vi "Data_Decimate.vi"(5 "Decimate ?":bool, 7 "Is Mass ?":bool, 8 "error in (no error)":errorcluster, 10 "Dataset":cluster{sgl[], sgl[]}[](array[cluster]), 11 "GraphXY":refnum<vi>) -> (0 "error out":errorcluster)   [LabVIEW 2018]
doc: "This VI decimates the data for the GraphXY.\n- Checks the X-scale of the GraphXY, the size of the data, and the pixel size of the screen\n- If the size of the data to be diplayed is less than 1 million of pixels : do nothing\n- If the size of the data is too large for the current display, decimate the data\n- The decimation factor is function of the \"Points per Pixel\" multiplied by the size of the screen in pixels\n- The \"Points per Pixel\" value can be updated through the global variable \"GraphXY Points per Pixel\""
uses:
  Global_Variables.vi
panel:
  out "Number of Points Currently Displayed":i32
  out "Decimation Factor":u32
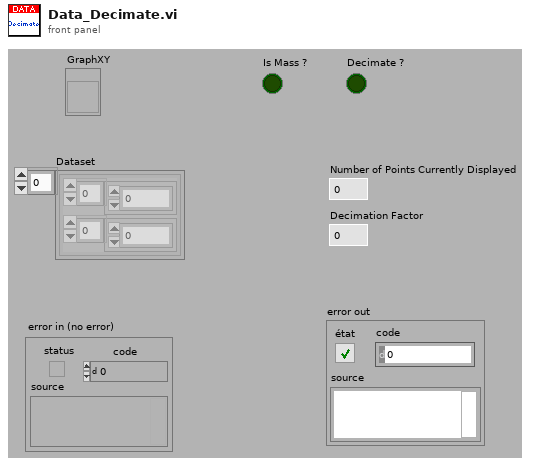
[diagram p1: front panel]
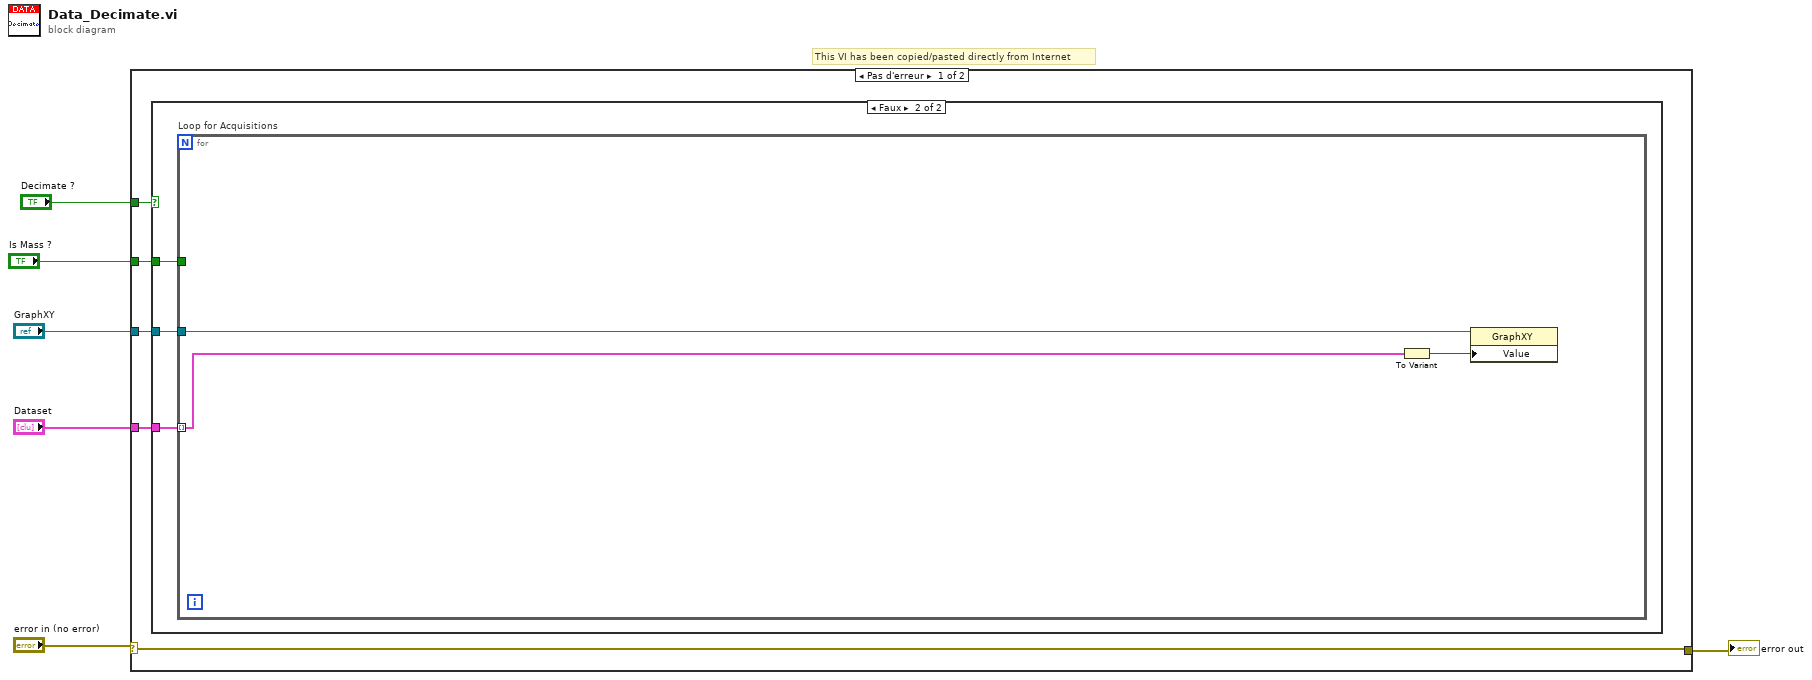
[diagram p0: block diagram]
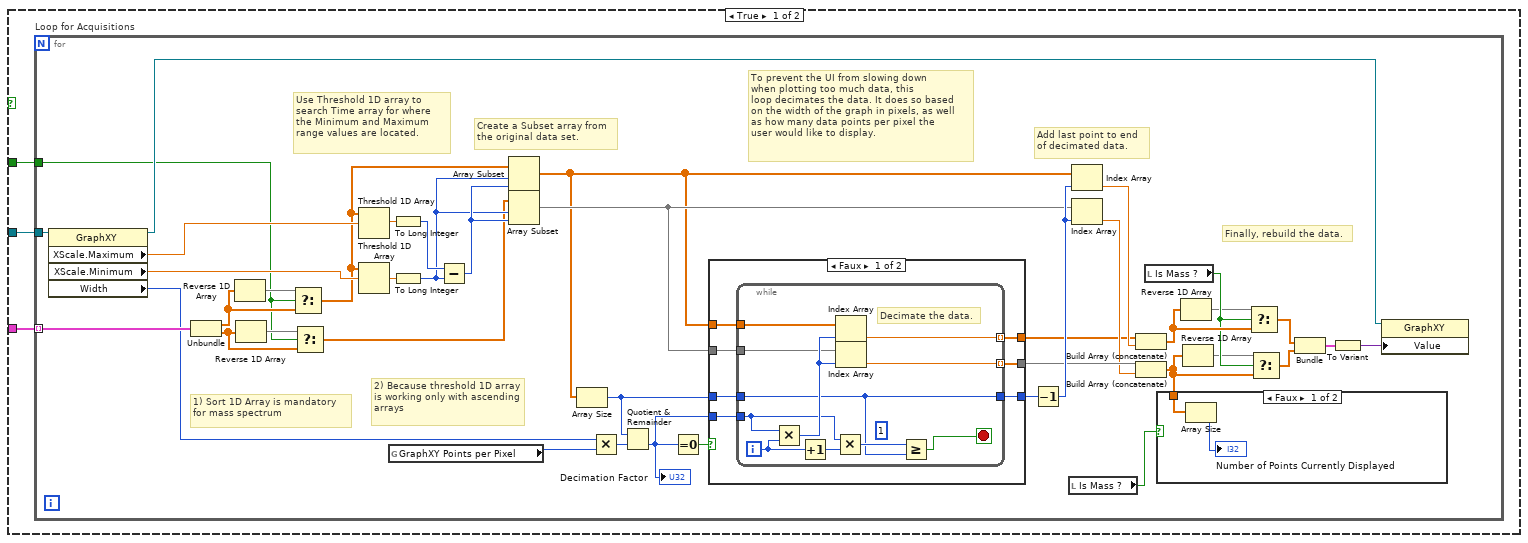
[diagram p2: hidden frame]
diagram:
  # "This VI has been copied/pasted directly from Internet"
  n1 = case shown="Pas d'erreur" "error in (no error)" {
    selector: "error in (no error)" -> [w9 w85]
    tunnel: [w9 w85] -> w5
    tunnel: "GraphXY" -> [w10 _]
    tunnel: "Dataset" -> [w11 _]
    tunnel: "Is Mass ?" -> [w8 _]
    tunnel: "Decimate ?" -> [w7 _]
    frame No Error {
      n2 = case shown="Faux" w7 {
        tunnel: w11 -> [w14 w81]
        tunnel: w10 -> [w13 w80]
        tunnel: w8 -> [w12 w79]
        frame True {
          n3 = for "Loop for Acquisitions" {
            tunnel: w14 -> [w55] mode=indexing
            tunnel: w13 -> [w54]
            tunnel: w12 -> [w23]
            # "1) Sort 1D Array is mandatory for mass spectrum"
            # "2) Because threshold 1D array is working only with ascending arrays"
            # "Add last point to end\nof decimated data."
            # "Finally, rebuild the data."
            # "To prevent the UI from slowing down\nwhen plotting too much data, this\nloop decimates the data. It does so based\non the width of the graph in pixels, as well\nas how many data points per pixel the\nuser would like to display."
            # "Create a Subset array from\nthe original data set."
            # "Use Threshold 1D array to\nsearch Time array for where\nthe Minimum and Maximum\nrange values are located."
            n4 = property class="GraphXY"(reference=w54) -> (reference out=w31:refnum<vi>, "XScale.Maximum"=w36:dbl, "XScale.Minimum"=w35:dbl, "Width"=w32:u32)  [unwired: 1 in, 1 out]
            n5 = Unbundle(w55) -> (w29:sgl[], w24:sgl[])
            n6 = Reverse 1D Array(array=w29) -> (reversed array=w28:sgl[])
            n7 = Reverse 1D Array(array=w24) -> (reversed array=w26:sgl[])
            n8 = Select(t=w28, s=w23, f=w29) -> (s? t:f=w27:sgl[])
            n9 = Select(t=w26, s=w23, f=w24) -> (s? t:f=w25:sgl[])
            n10 = Threshold 1D Array(2:w36, 3:w27) -> (0:w52:sgl)  [unwired: 1 in]
            n11 = Threshold 1D Array(2:w35, 3:w27) -> (0:w51:sgl)  [unwired: 1 in]
            n12 = global read "Global_Variables.vi" "GraphXY Points per Pixel"() -> (w30:i32)
            n13 = To Long Integer(number=w52) -> (32bit integer=w44:i32)
            n14 = To Long Integer(number=w51) -> (32bit integer=w43:i32)
            n15 = Subtract(x=w44, y=w43) -> (x-y=w53:i32)
            n16 = Array Subset(array=w27, index=w43, length=w53) -> (w38:sgl[])
            n17 = Array Subset(array=w25, index=w43, length=w53) -> (w48:sgl[])
            n18 = Array Size(array=w38) -> (size(s)=w42:i32)
            n19 = Multiply(x=w32, y=w30) -> (x*y=w39:u32)
            n20 = Quotient & Remainder(x=w42, y=w39) -> (floor(x/y)=w37:u32)  [unwired: 1 out]
            "Decimation Factor" <- w37
            n21 = Equal To 0?(x=w37) -> (x = 0?=w40:bool)
            n22 = case shown="Faux" w40 {
              tunnel: [w64 w76] -> w50
              tunnel: w38 -> [w63 w78]
              tunnel: w48 -> [w62 w77]
              tunnel: [w61 w77] -> w47
              tunnel: w42 -> [w60 w76]
              tunnel: [w59 w78] -> w41
              tunnel: w37 -> [w58 _]
              frame False {
                n23 = while {
                  tunnel: w63 -> [w72]
                  tunnel: w62 -> [w68]
                  tunnel: w60 -> [w66]
                  tunnel: [w70] -> w59 mode=indexing
                  tunnel: [w69] -> w61 mode=indexing
                  tunnel: w58 -> [w67]
                  tunnel: [w66] -> w64
                  i -> [w75]
                  stop <- w65 stop-if-true
                  (unwired) u32 1 ("y")
                  # "Decimate the data."
                  n24 = Multiply(x=w67, y=w75) -> (x*y=w71:u32)
                  n25 = Increment(x=w75) -> (x+1=w74:i32)
                  n26 = Multiply(x=w67, y=w74) -> (x*y=w73:u32)
                  n27 = Index Array(array=w72, index=w71) -> (element=w70:sgl)
                  n28 = Index Array(array=w68, index=w71) -> (element=w69:sgl)
                  n29 = Greater Or Equal?(x=w73, y=w66) -> (x >= y?=w65:bool)
                }
              }
              frame True {
              }
            }
            n30 = Decrement(x=w50) -> (x-1=w49:i32)
            n31 = local read "Is Mass ?"() -> (w15:bool)
            n32 = Index Array(array=w38, index=w49) -> (element=w45:sgl)
            n33 = Index Array(array=w48, index=w49) -> (element=w46:sgl)
            n34 = Build Array (concatenate)(w41, w45) -> (w20:sgl[])
            n35 = Build Array (concatenate)(w47, w46) -> (w16:sgl[])
            n36 = local read "Is Mass ?"() -> (w19:bool)
            n37 = case shown="Faux" w15 {
              tunnel: w16 -> [w56 _]
              frame False {
                n38 = Array Size(array=w56) -> (size(s)=→"Number of Points Currently Displayed":i32)
              }
              frame True {
              }
            }
            n39 = Reverse 1D Array(array=w20) -> (reversed array=w18:sgl[])
            n40 = Reverse 1D Array(array=w16) -> (reversed array=w17:sgl[])
            n41 = Select(t=w18, s=w19, f=w20) -> (s? t:f=w22:sgl[])
            n42 = Select(t=w17, s=w19, f=w16) -> (s? t:f=w21:sgl[])
            n43 = Bundle(w22, w21) -> (w33:cluster{sgl[], sgl[]})  [unwired: 1 in]
            n44 = To Variant(anything=w33) -> (Variant=w34:variant)
            n45 = property class="GraphXY"(reference=w31, "Value"=w34) -> ()  [unwired: 1 in, 2 out]
          }
        }
        frame False {
          n46 = for "Loop for Acquisitions" {
            tunnel: w81 -> [w83] mode=indexing
            tunnel: w80 -> [w84]
            tunnel: w79 -> [_]
            n47 = To Variant(anything=w83) -> (Variant=w82:variant)
            n48 = property class="GraphXY"(reference=w84, "Value"=w82) -> ()  [unwired: 1 in, 2 out]
          }
        }
      }
    }
    frame Error {
    }
  }
  "error out" <- w5
